vi "未命名 17.vi"() -> (0 "error out":errorcluster caption="错误输出", 3 "task out":refnum<k21> caption="任务输出")   [LabVIEW 2020]
uses:
  <vilib>/DAQmx/create/channels.llb/DAQmx Create Channel (CI-Position-Angular Encoder).vi
  <resource>/objmgr/daqmx.rc
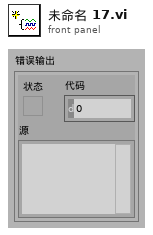
[diagram p1: front panel]
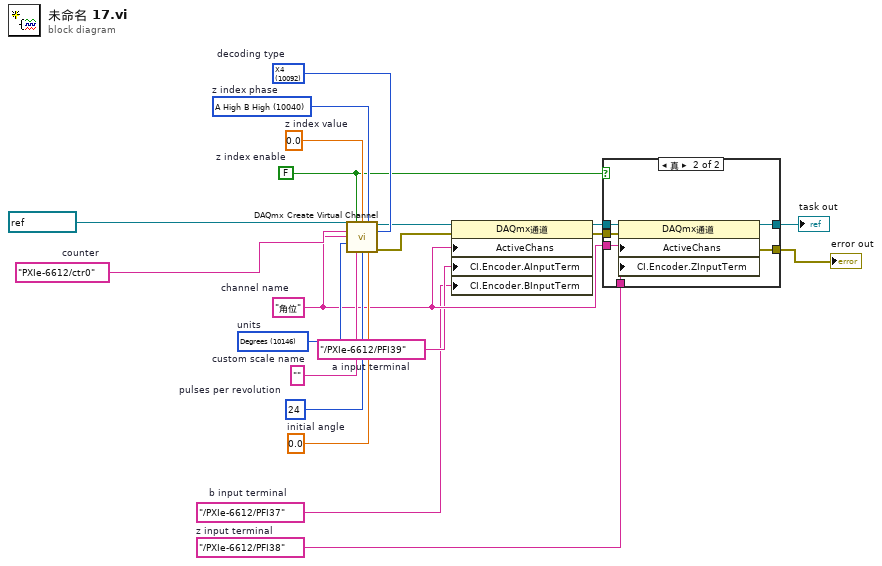
[diagram p0: block diagram]
diagram:
  w2 = "/PXIe-6612/PFI38"  # z input terminal
  w3 = "/PXIe-6612/PFI37"  # b input terminal
  w4 = "/PXIe-6612/PFI39"  # a input terminal
  w16 = 10146 items=["Degrees"=10146, "Radians"=10273, "Ticks"=10304, "From Custom Scale"=10065]  # units
  w12 = 10092 items=["X1"=10090, "X2"=10091, "X4"=10092, "Two Pulse Counting"=10313]  # decoding type
  w13 = 0.0  # initial angle
  w14 = u32 24  # pulses per revolution
  w15 = ""  # custom scale name
  w17 = 10040 items=["A High B High"=10040, "A High B Low"=10041, "A Low B High"=10042, "A Low B Low"=10043]  # z index phase
  w18 = 0.0  # z index value
  w6 = FALSE  # z index enable
  w5 = "角位"  # channel name
  w20 = "PXIe-6612/ctr0"  # counter
  n1 = call-poly <vilib>:"DAQmx Create Virtual Channel.vi"("task in"=refnum<k21> "6612-0", "z index enable"=w6, "z index value"=w18, "z index phase"=w17, "counter"=w20, "decoding type"=w12, "name to assign"=w5, "units"=w16, "custom scale name"=w15, "pulses per revolution"=w14, "initial angle"=w13) -> ("task out"=w11:refnum<k21>, "error out"=w19:errorcluster)  [unwired: 3 in]
  n2 = property class="DAQmx通道"(reference=w11, error in=w19, "ActiveChans"=w5, "CI.Encoder.AInputTerm"=w4, "CI.Encoder.BInputTerm"=w3) -> (reference out=w10:refnum<k21>, error out=w9:errorcluster)
  n3 = case "条件结构" shown="真" w6 {
    tunnel: w10 -> [w22 w28]
    tunnel: w9 -> [w21 w27]
    tunnel: [w22 w26] -> w8
    tunnel: [w21 w25] -> w7
    tunnel: w5 -> [_ w24]
    tunnel: w2 -> [_ w23]
    frame False {
    }
    frame True {
      n4 = property class="DAQmx通道"(reference=w28, error in=w27, "ActiveChans"=w24, "CI.Encoder.ZInputTerm"=w23) -> (reference out=w26:refnum<k21>, error out=w25:errorcluster)
    }
  }
  "error out" <- w7
  "task out" <- w8
